vi "Analog Get Voltage.vi"(11 "Analog Channel":T1(ring)=enum."AI MXP 0") -> (3 "Voltage":dbl min=0.0 max=5.0)   [LabVIEW 2016]
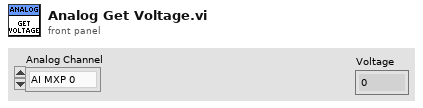
[diagram p1: front panel]
types:
  T1 = enum8{"AI 0", "AI 1", "AI 2", "AI 3", "AI MXP 0", "AI MXP 1", "AI MXP 2", "AI MXP 3", "Invalid"}
  T2 = typedef "WPI_AnalogChannelDevRef.ctl" = cluster{"DevStatus":errorcluster, "Analog Channel":T3}
  T3 = typedef "FPGA_AIChannel.ctl" = enum8{"AI 0", "AI 1", "AI 2", "AI 3", "AI MXP 0", "AI MXP 1", "AI MXP 2", "AI MXP 3", "Invalid"}
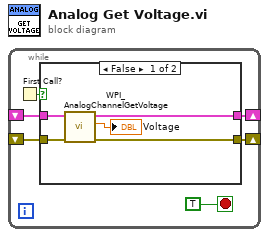
[diagram p0: block diagram]
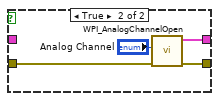
[diagram p2: hidden frame]
diagram:
  n1 = while {
    shift-right: [w5] -> _
    shift-left: _ -> [w4]
    shift-right: [w3] -> _
    shift-left: _ -> [w2]
    stop <- TRUE stop-if-true
    n2 = First Call?() -> (First Call?: T/F=w6:bool)
    n3 = case shown="False" w6 {
      tunnel: [w9 w15] -> w5
      tunnel: w4 -> [w11 w14]
      tunnel: [w10 w13] -> w3
      tunnel: w2 -> [w8 _]
      frame False {
        n4 = call <vilib>:"WPI_AnalogChannelGetVoltage.vi"("error in (no error)"=w11, "AIDeviceRef"=w8) -> ("error out"=w9:errorcluster, "Voltage"=→"Voltage":dbl, "AIDeviceRef"=w10:T2)  [unwired: 7 in]
      }
      frame True {
        n5 = call <vilib>:"WPI_AnalogChannelOpen.vi"("error in (no error)"=w14, "Analog Channel"="Analog Channel") -> ("error out"=w15:errorcluster, "AIDeviceRef"=w13:T2)  [unwired: 8 in]
      }
    }
  }
